vi "Calculate Modbus CRC16.vi"(1 "Data Bytes":string) -> (0 "Calculated CRC":u16 format="%x")   [LabVIEW 2026]
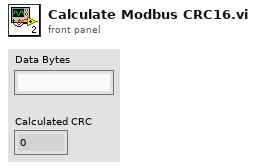
[diagram p1: front panel]
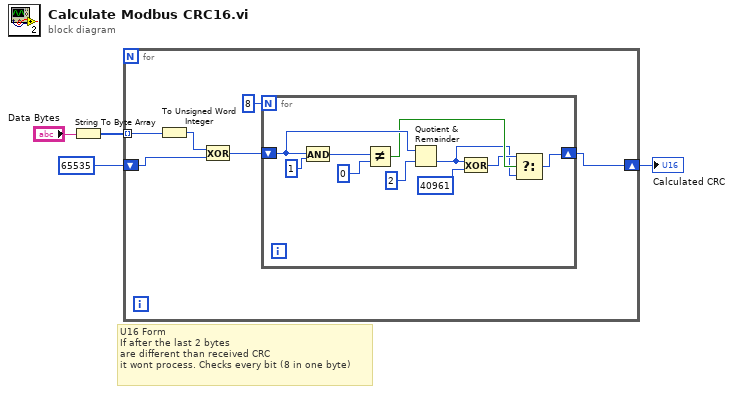
[diagram p0: block diagram]
diagram:
  # "U16 Form\nIf after the last 2 bytes\nare different than received CRC\nit wont process. Checks every bit (8 in one byte)"
  n1 = String To Byte Array(string="Data Bytes") -> (unsigned byte array=w3:u8[])
  n2 = for {
    tunnel: w3 -> [w9] mode=indexing
    shift-right: [w5] -> w1
    shift-left: u16 65535 -> [w6]
    n3 = To Unsigned Word Integer(number=w9) -> (unsigned 16bit integer=w10:u16)
    n4 = Exclusive Or(1:w6, 2:w10) -> (0:w7:u16)
    n5 = for {
      N: 8 -> [_]
      shift-right: [w14] -> w5
      shift-left: w7 -> [w17]
      n6 = And(x=w17, y=u16 1) -> (x .and. y?=w18:u16)
      n7 = Not Equal?(x=w18, y=u16 0) -> (x != y?=w13:bool)
      n8 = Quotient & Remainder(x=w17, y=u16 2) -> (floor(x/y)=w11:u16)  [unwired: 1 out]
      n9 = Exclusive Or(1:u16 40961 ("y"), 2:w11) -> (0:w12:u16)
      n10 = Select(t=w12, s=w13, f=w11) -> (s? t:f=w14:u16)
    }
  }
  "Calculated CRC" <- w1
